vi "Hide.vi"(8 "error in (no error)":errorcluster, 11 "SMO.UI":refnum<class "SMO.UI.lvclass">) -> (0 "error out":errorcluster, 3 "SMO.UI out":refnum<class "SMO.UI.lvclass">)   [LabVIEW 2013, in "SMO.UI.lvclass"]
doc: "Close the front panel of the SMO.UI. \nNote that this method does not stop the Process.vi."
uses:
  SMO.UI.lvclass
panel:
  # "For instructions on how to use the JKI State Machine Objects, examples and video tutorials, visit:\nhttp://jki.net/state-machine-objects/\n\nJKI State Machine Objects™\nhttp://jki.net/state-machine-objects/\nCopyright (C) 2005-2015, JKI <info@jki.net>\nALL RIGHTS RESERVED"
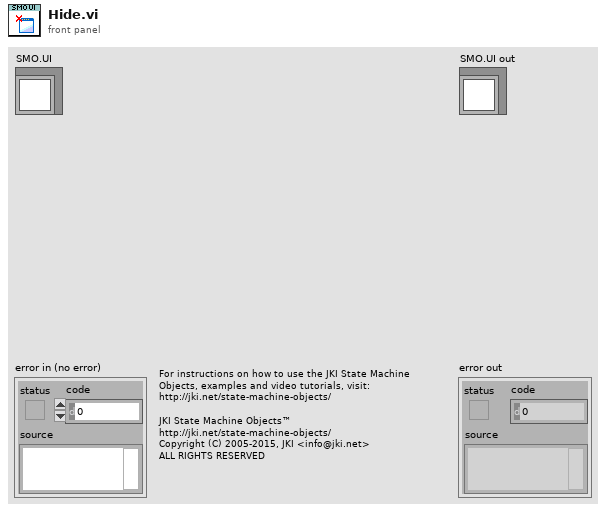
[diagram p1: front panel]
types:
  T1 = typedef "SMO.UI.lvclass/PrivateEvents--Cluster.ctl" = cluster{"Show-Hide UI":refnum<user-event>}
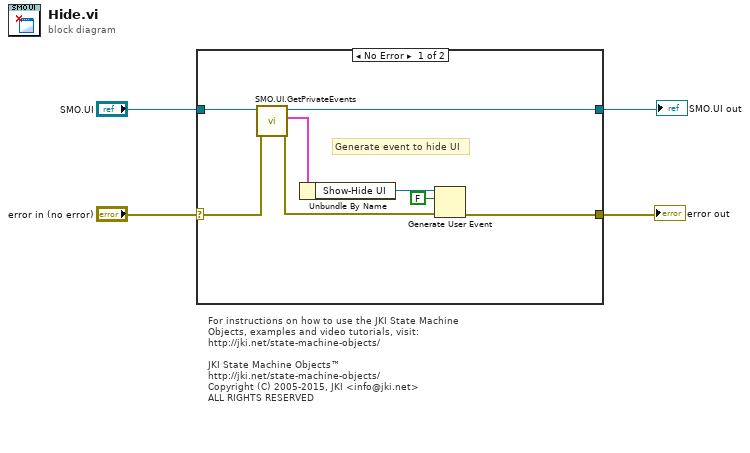
[diagram p0: block diagram]
diagram:
  # "For instructions on how to use the JKI State Machine Objects, examples and video tutorials, visit:\nhttp://jki.net/state-machine-objects/\n\nJKI State Machine Objects™\nhttp://jki.net/state-machine-objects/\nCopyright (C) 2005-2015, JKI <info@jki.net>\nALL RIGHTS RESERVED"
  n1 = case shown="No Error" "error in (no error)" {
    selector: "error in (no error)" -> [w5 w14]
    tunnel: "SMO.UI" -> [w7 w13]
    tunnel: [w6 w14] -> w1
    tunnel: [w12 w13] -> w2
    frame No Error {
      # "Generate event to hide UI"
      n2 = call "SMO.UI.GetPrivateEvents.vi"("error in (no error)"=w5, "SMO.UI"=w7) -> ("error out"=w11:errorcluster, "SMO.UI Private Events"=w9:T1, "SMO.UI out"=w12:refnum<class "SMO.UI.lvclass">)  [unwired: 7 in]
      n3 = Unbundle By Name(w9) -> ("Show-Hide UI"=w10:refnum<user-event>)
      n4 = Generate User Event(user event=w10, event data cluster=FALSE ("event data"), error in=w11) -> (error out=w6:errorcluster)  [unwired: 1 in, 1 out]
    }
    frame Error {
    }
  }
  "error out" <- w1
  "SMO.UI out" <- w2
